vi "loadHTMLHist.vi"() -> ()   [LabVIEW 2012]
uses:
  <vilib>/addons/database/Connection.llb/DB Tools Open Connec (Path).vi
  <vilib>/addons/database/NI_Database_API.lvlib
panel:
  out "error out":errorcluster
  in  "input cluster 2":T1
  in  "error in (no error)":errorcluster
  out "filenames":string[](array[string])
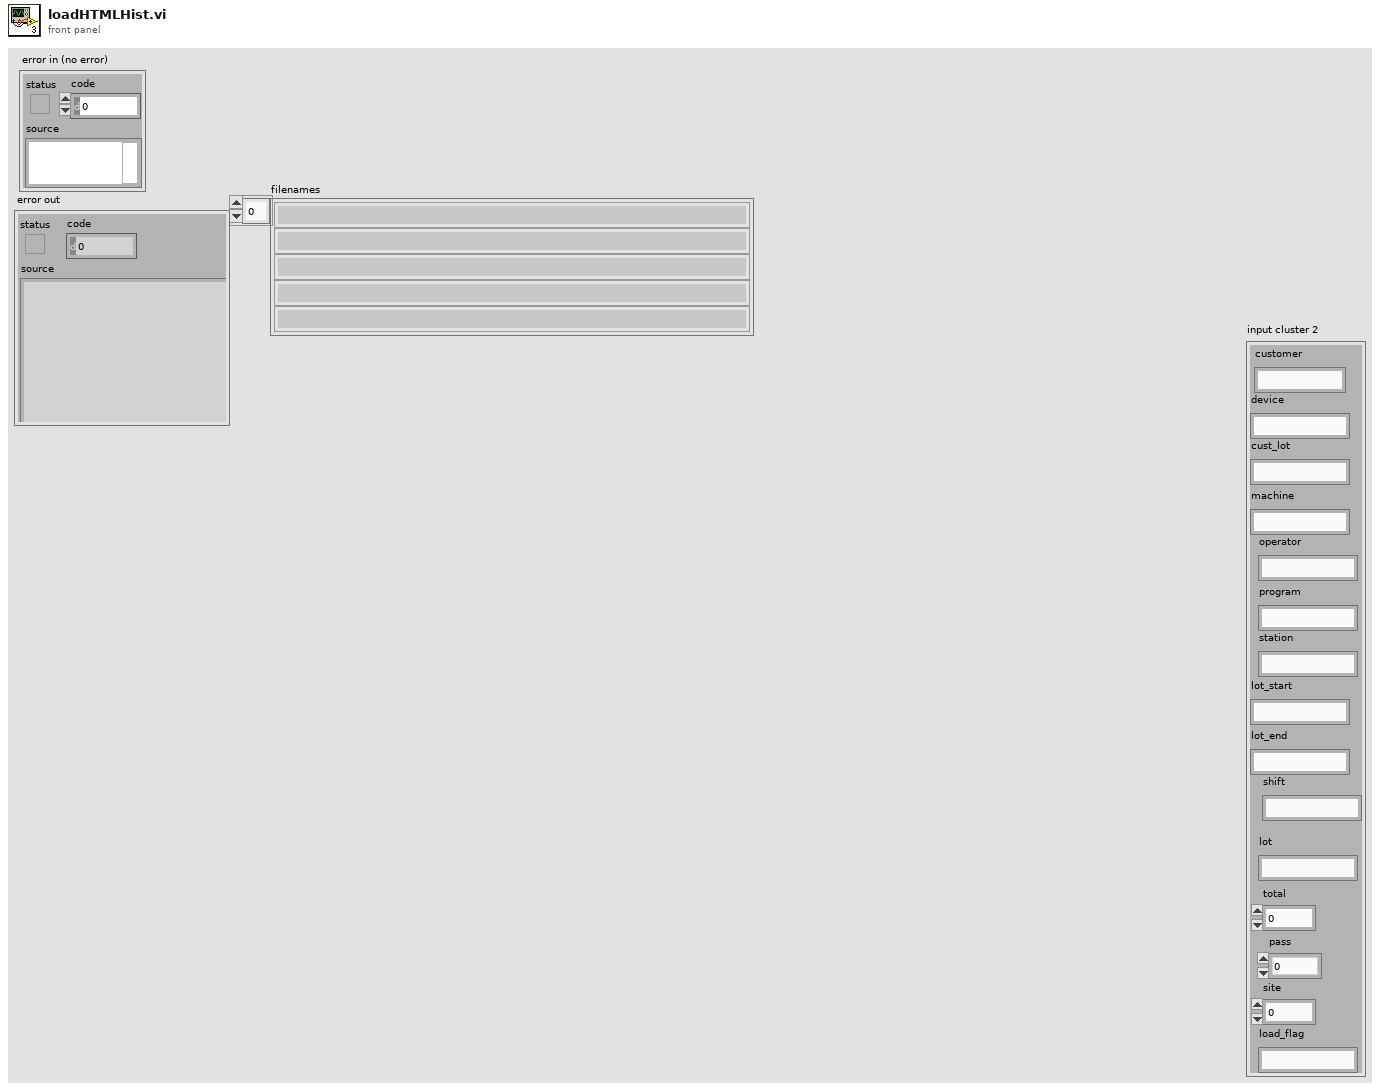
[diagram p1: front panel]
types:
  T1 = cluster{"customer":string, "device":string, "cust_lot":string, "machine":string, "operator":string, "program":string, "station":string, "lot_start":string, "lot_end":string, "shift":string, "lot":string, "total":dbl, "pass":dbl, "load_flag":string, "site":dbl}
  T2 = typedef "NI_Database_API.lvlib/Conn ObjectReference.ctl" = refnum<k1>
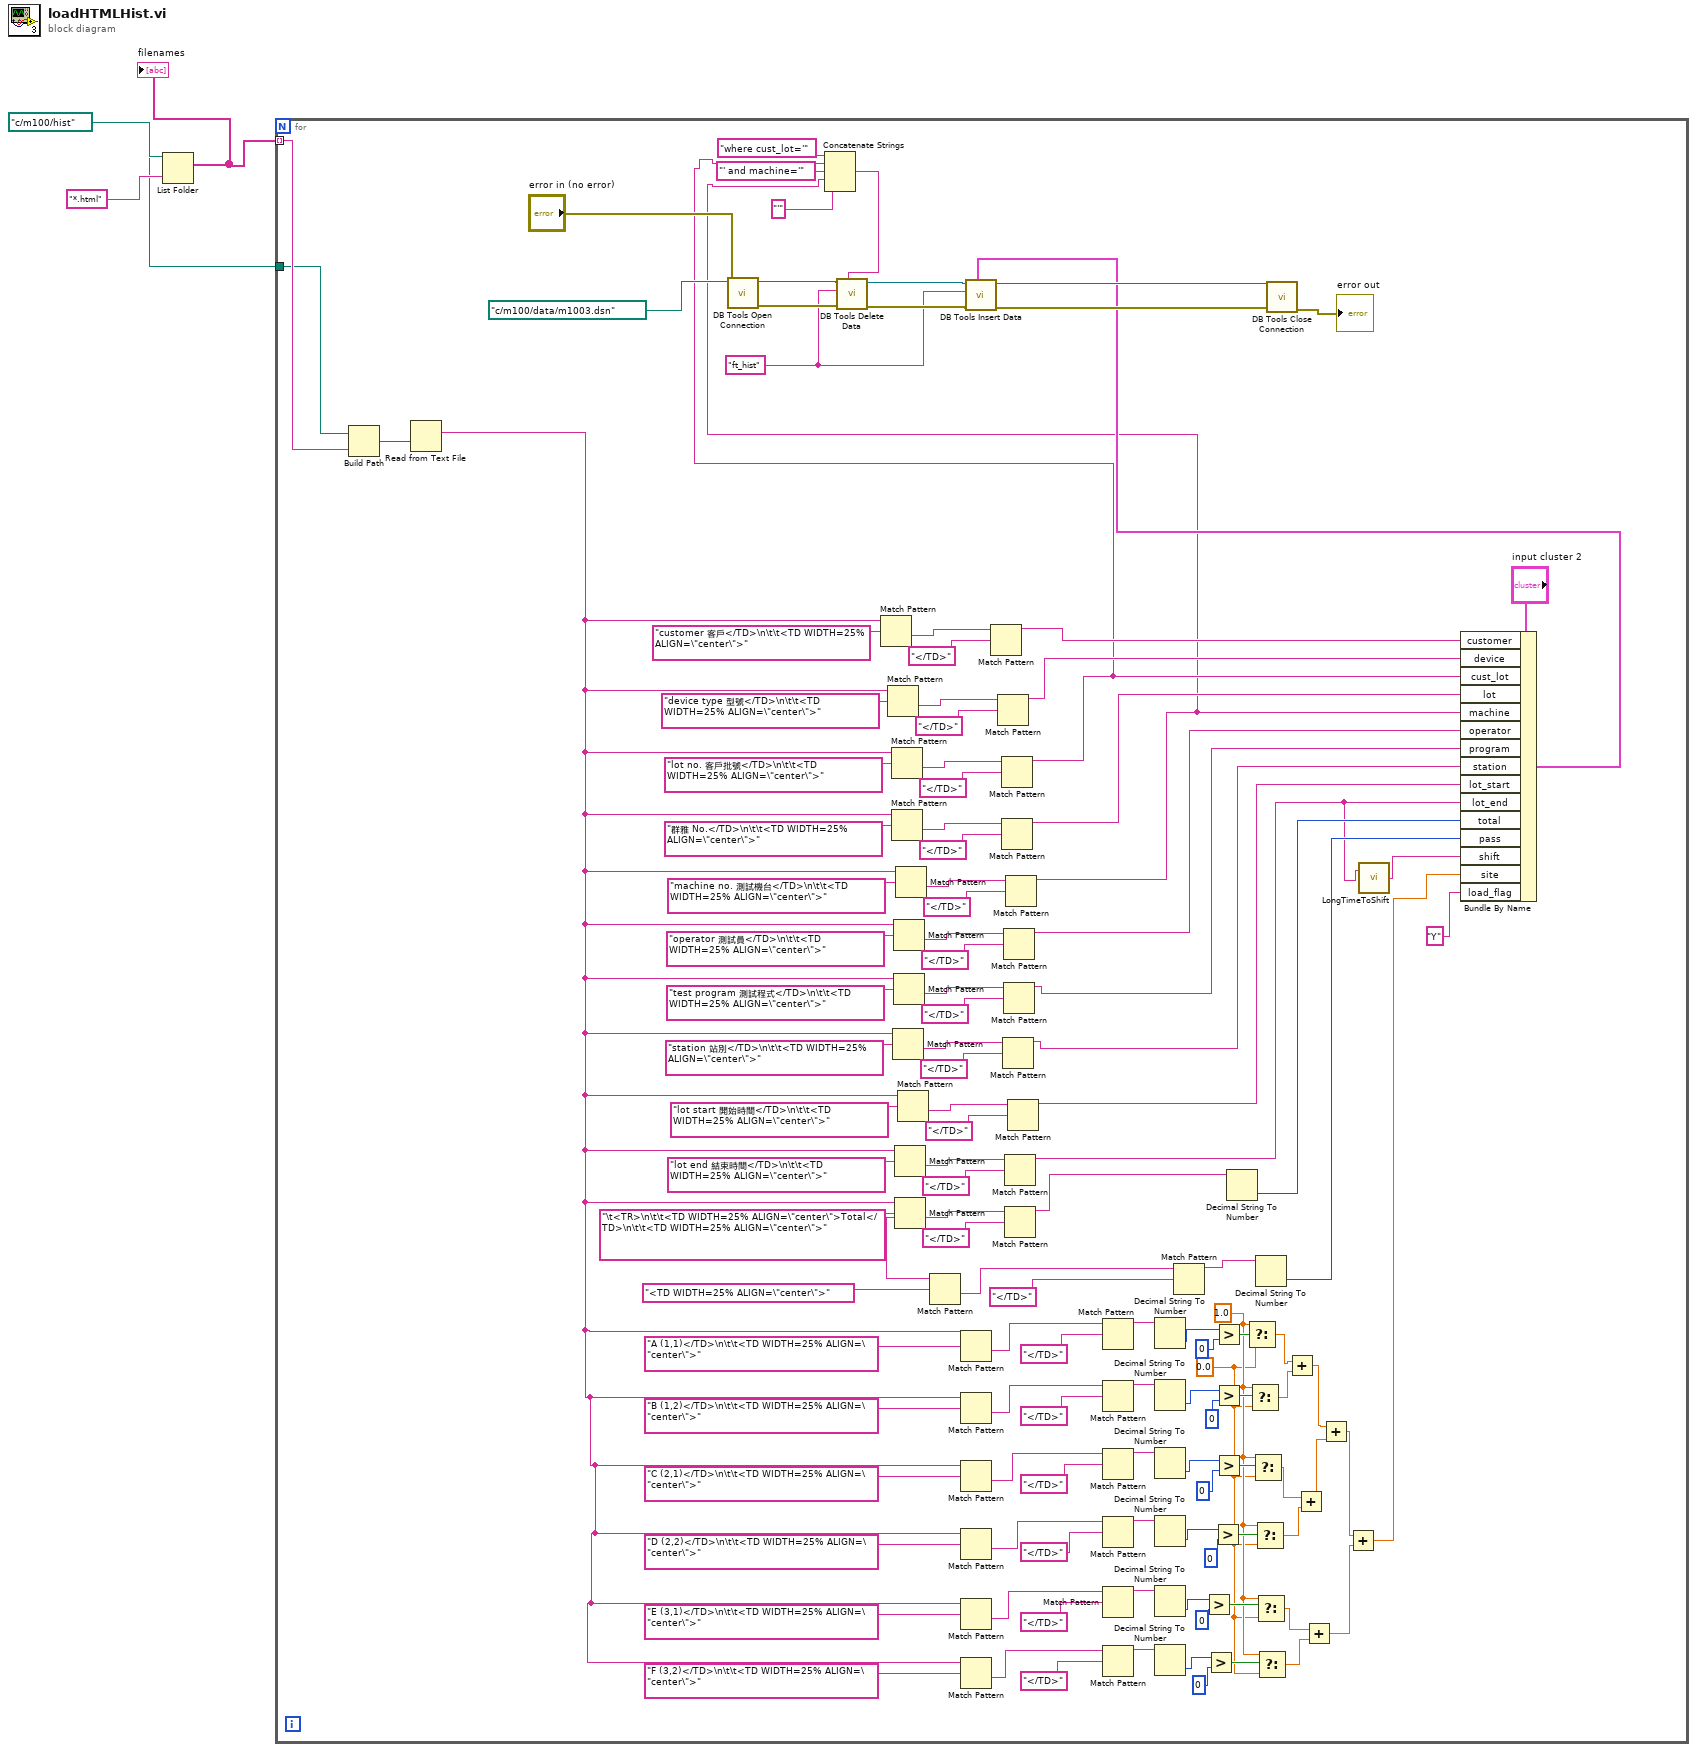
[diagram p0: block diagram]
diagram:
  n1 = List Folder(path=path "c:/m100/hist", pattern="*.html") -> (path out=w1:path, filenames=w2:string[])  [unwired: 2 in, 2 out]
  "filenames" <- w2
  n2 = for {
    tunnel: w2 -> [w129] mode=indexing
    tunnel: w1 -> [w128]
    w23 = 0.0 ("f")
    w24 = 1.0 ("t")
    w69 = "ft_hist" ("table 2")
    n3 = Build Path(base path=w128, name or relative path=w129) -> (appended path=w130:path)
    n4 = Read from Text File(file (use dialog)=w130) -> (text=w37:string)  [unwired: 3 in, 3 out]
    n5 = call-poly <vilib>:"DB Tools Open Connection.vi"("error in (no error)"="error in (no error)", "connection information"=path "c:/m100/data/m1003.dsn") -> ("error out"=w71:errorcluster, "connection reference"=w73:T2)  [unwired: 6 in]
    n6 = Match Pattern(string=w37, regular expression="customer 客戶</TD>\n\t\t<TD WIDTH=25% ALIGN=\"center\">") -> (after substring=w126:string)  [unwired: 1 in, 3 out]
    n7 = Match Pattern(string=w37, regular expression="device type 型號</TD>\n\t\t<TD WIDTH=25% ALIGN=\"center\">") -> (after substring=w123:string)  [unwired: 1 in, 3 out]
    n8 = Match Pattern(string=w37, regular expression="lot no. 客戶批號</TD>\n\t\t<TD WIDTH=25% ALIGN=\"center\">") -> (after substring=w120:string)  [unwired: 1 in, 3 out]
    n9 = Match Pattern(string=w37, regular expression="群雅 No.</TD>\n\t\t<TD WIDTH=25% ALIGN=\"center\">") -> (after substring=w117:string)  [unwired: 1 in, 3 out]
    n10 = Match Pattern(string=w37, regular expression="station 站別</TD>\n\t\t<TD WIDTH=25% ALIGN=\"center\">") -> (after substring=w105:string)  [unwired: 1 in, 3 out]
    n11 = Match Pattern(string=w37, regular expression="operator 測試員</TD>\n\t\t<TD WIDTH=25% ALIGN=\"center\">") -> (after substring=w111:string)  [unwired: 1 in, 3 out]
    n12 = Match Pattern(string=w37, regular expression="test program 測試程式</TD>\n\t\t<TD WIDTH=25% ALIGN=\"center\">") -> (after substring=w108:string)  [unwired: 1 in, 3 out]
    n13 = Match Pattern(string=w37, regular expression="lot end 結束時間</TD>\n\t\t<TD WIDTH=25% ALIGN=\"center\">") -> (after substring=w99:string)  [unwired: 1 in, 3 out]
    n14 = Match Pattern(string=w37, regular expression="\t<TR>\n\t\t<TD WIDTH=25% ALIGN=\"center\">Total</TD>\n\t\t<TD WIDTH=25% ALIGN=\"center\">") -> (after substring=w95:string)  [unwired: 1 in, 3 out]
    n15 = Match Pattern(string=w37, regular expression="machine no. 測試機台</TD>\n\t\t<TD WIDTH=25% ALIGN=\"center\">") -> (after substring=w114:string)  [unwired: 1 in, 3 out]
    n16 = Match Pattern(string=w37, regular expression="lot start 開始時間</TD>\n\t\t<TD WIDTH=25% ALIGN=\"center\">") -> (after substring=w102:string)  [unwired: 1 in, 3 out]
    n17 = Match Pattern(string=w95, regular expression="<TD WIDTH=25% ALIGN=\"center\">") -> (after substring=w92:string)  [unwired: 1 in, 3 out]
    n18 = Match Pattern(string=w37, regular expression="A (1,1)</TD>\n\t\t<TD WIDTH=25% ALIGN=\"center\">") -> (after substring=w60:string)  [unwired: 1 in, 3 out]
    n19 = Match Pattern(string=w37, regular expression="B (1,2)</TD>\n\t\t<TD WIDTH=25% ALIGN=\"center\">") -> (after substring=w55:string)  [unwired: 1 in, 3 out]
    n20 = Match Pattern(string=w37, regular expression="C (2,1)</TD>\n\t\t<TD WIDTH=25% ALIGN=\"center\">") -> (after substring=w51:string)  [unwired: 1 in, 3 out]
    n21 = Match Pattern(string=w37, regular expression="D (2,2)</TD>\n\t\t<TD WIDTH=25% ALIGN=\"center\">") -> (after substring=w47:string)  [unwired: 1 in, 3 out]
    n22 = Match Pattern(string=w37, regular expression="E (3,1)</TD>\n\t\t<TD WIDTH=25% ALIGN=\"center\">") -> (after substring=w43:string)  [unwired: 1 in, 3 out]
    n23 = Match Pattern(string=w37, regular expression="F (3,2)</TD>\n\t\t<TD WIDTH=25% ALIGN=\"center\">") -> (after substring=w39:string)  [unwired: 1 in, 3 out]
    n24 = Match Pattern(string=w126, regular expression="</TD>") -> (before substring=w88:string)  [unwired: 1 in, 3 out]
    n25 = Match Pattern(string=w123, regular expression="</TD>") -> (before substring=w87:string)  [unwired: 1 in, 3 out]
    n26 = Match Pattern(string=w120, regular expression="</TD>") -> (before substring=w67:string)  [unwired: 1 in, 3 out]
    n27 = Match Pattern(string=w117, regular expression="</TD>") -> (before substring=w86:string)  [unwired: 1 in, 3 out]
    n28 = Match Pattern(string=w105, regular expression="</TD>") -> (before substring=w83:string)  [unwired: 1 in, 3 out]
    n29 = Match Pattern(string=w111, regular expression="</TD>") -> (before substring=w85:string)  [unwired: 1 in, 3 out]
    n30 = Match Pattern(string=w108, regular expression="</TD>") -> (before substring=w84:string)  [unwired: 1 in, 3 out]
    n31 = Match Pattern(string=w99, regular expression="</TD>") -> (before substring=w79:string)  [unwired: 1 in, 3 out]
    n32 = Match Pattern(string=w95, regular expression="</TD>") -> (before substring=w91:string)  [unwired: 1 in, 3 out]
    n33 = Match Pattern(string=w114, regular expression="</TD>") -> (before substring=w65:string)  [unwired: 1 in, 3 out]
    n34 = Concatenate Strings("where cust_lot='" ("string"), w67, "' and machine='" ("string"), w65, "'" ("string")) -> (w63:string)
    n35 = call <vilib>:"DB Tools Delete Data.vi"("condition"=w63, "error in (no error)"=w71, "table"=w69, "connection reference"=w73) -> ("error out"=w70:errorcluster, "connection reference out"=w72:T2)  [unwired: 6 in]
    n36 = Match Pattern(string=w102, regular expression="</TD>") -> (before substring=w82:string)  [unwired: 1 in, 3 out]
    n37 = Match Pattern(string=w60, regular expression="</TD>") -> (before substring=w58:string)  [unwired: 1 in, 3 out]
    n38 = Match Pattern(string=w55, regular expression="</TD>") -> (before substring=w54:string)  [unwired: 1 in, 3 out]
    n39 = Match Pattern(string=w51, regular expression="</TD>") -> (before substring=w50:string)  [unwired: 1 in, 3 out]
    n40 = Match Pattern(string=w47, regular expression="</TD>") -> (before substring=w46:string)  [unwired: 1 in, 3 out]
    n41 = Match Pattern(string=w43, regular expression="</TD>") -> (before substring=w42:string)  [unwired: 1 in, 3 out]
    n42 = Match Pattern(string=w39, regular expression="</TD>") -> (before substring=w38:string)  [unwired: 1 in, 3 out]
    n43 = Decimal String To Number(string=w58) -> (number=w8:i32)  [unwired: 2 in, 1 out]
    n44 = Decimal String To Number(string=w54) -> (number=w9:i32)  [unwired: 2 in, 1 out]
    n45 = Decimal String To Number(string=w50) -> (number=w10:i32)  [unwired: 2 in, 1 out]
    n46 = Decimal String To Number(string=w46) -> (number=w11:i32)  [unwired: 2 in, 1 out]
    n47 = Decimal String To Number(string=w42) -> (number=w12:i32)  [unwired: 2 in, 1 out]
    n48 = Decimal String To Number(string=w38) -> (number=w7:i32)  [unwired: 2 in, 1 out]
    n49 = Match Pattern(string=w92, regular expression="</TD>") -> (before substring=w59:string)  [unwired: 1 in, 3 out]
    n50 = Greater?(x=w12, y=0) -> (0:w26:bool)
    n51 = Greater?(x=w7, y=0) -> (0:w25:bool)
    n52 = Greater?(x=w11, y=0) -> (0:w27:bool)
    n53 = Greater?(x=w8, y=0) -> (0:w30:bool)
    n54 = Greater?(x=w9, y=0) -> (0:w29:bool)
    n55 = Greater?(x=w10, y=0) -> (0:w28:bool)
    n56 = Decimal String To Number(string=w91) -> (number=w81:i32)  [unwired: 2 in, 1 out]
    n57 = Select(t=w24, s=w30, f=w23) -> (s? t:f=w21:dbl)
    n58 = Select(t=w24, s=w29, f=w23) -> (s? t:f=w22:dbl)
    n59 = Select(t=w24, s=w28, f=w23) -> (s? t:f=w20:dbl)
    n60 = Select(t=w24, s=w27, f=w23) -> (s? t:f=w19:dbl)
    n61 = Decimal String To Number(string=w59) -> (number=w80:i32)  [unwired: 2 in, 1 out]
    n62 = Select(t=w24, s=w26, f=w23) -> (s? t:f=w18:dbl)
    n63 = Select(t=w24, s=w25, f=w23) -> (s? t:f=w17:dbl)
    n64 = Add(x=w21, y=w22) -> (x+y=w15:dbl)
    n65 = Add(x=w20, y=w19) -> (x+y=w16:dbl)
    n66 = Add(x=w18, y=w17) -> (x+y=w14:dbl)
    n67 = Add(x=w15, y=w16) -> (x+y=w13:dbl)
    n68 = Add(x=w13, y=w14) -> (x+y=w5:dbl)
    n69 = call "LongTimeToShift.vi"("input string"=w79) -> ("s? t:f"=w78:string)  [unwired: 1 in]
    n70 = Bundle By Name(cluster="input cluster 2", "customer"=w88, "device"=w87, "cust_lot"=w67, "lot"=w86, "machine"=w65, "operator"=w85, "program"=w84, "station"=w83, "lot_start"=w82, "lot_end"=w79, "total"=w81, "pass"=w80, "shift"=w78, "site"=w5, "load_flag"="Y") -> (w75:T1)
    n71 = call <vilib>:"DB Tools Insert Data.vi"("data"=w75, "error in (no error)"=w70, "table"=w69, "connection reference"=w72) -> ("error out"=w76:errorcluster, "connection reference out"=w77:T2)  [unwired: 6 in]
    n72 = call <vilib>:"DB Tools Close Connection.vi"("error in (no error)"=w76, "connection reference"=w77) -> ("error out"=→"error out":errorcluster)  [unwired: 5 in]
  }
